vi "ClimbExecute.vi"(8 "error in (no error)":errorcluster) -> (0 "error out":errorcluster)   [LabVIEW 2023]
uses:
  <vilib>/Rock Robotics/WPI/ThirdParty/JAS_Junk/TrajLib/VI/BoolCmd_Recv_Internal.vi
  <vilib>/Rock Robotics/WPI/ThirdParty/JAS_Junk/TrajLib/VI/BoolCmd_ObtainQueue.vi
  <vilib>/Rock Robotics/Network Tables/NT Write Number.vi
  <vilib>/Rock Robotics/Network Tables/NT Write Boolean.vi
  <vilib>/Rock Robotics/WPI/ThirdParty/JAS_Junk/TrajLib/Trajectory_Library.lvlib
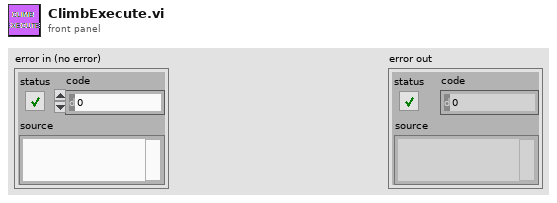
[diagram p1: front panel]
types:
  T1 = typedef "WPI_MotorControlDeviceRef.ctl" = cluster{"DeviceStatus":errorcluster, "Type":T2, "PWM":cluster{"PWM Channel":T3, "DeadBand":T4}, "CAN":cluster{"Device Number":u8, "SetOutput VI Ref":variant, "GetOutput VI Ref":variant, "Enable VI Ref":variant, "Disable VI Ref":variant, "Data":variant}, "Invert":bool, "DIO PWM":cluster{"PWM \"Enable\" Channel":T3, "DIOChannel":T5, "PWM Rate":dbl}}
  T2 = typedef "WPI_MotorControlType.ctl" = enum16{"PWM", "CAN", "DIO PWM"}
  T3 = typedef "FPGA_DIOPWMChannel.ctl" = enum8{"PWM 0", "PWM 1", "PWM 2", "PWM 3", "PWM 4", "PWM 5", "PWM 6", "PWM 7", "PWM 8", "PWM 9", "PWM MXP 0", "PWM MXP 1", "PWM MXP 2", "PWM MXP 3", "PWM MXP 4", "PWM MXP 5", "PWM MXP 6", "PWM MXP 7", "PWM MXP 8", "PWM MXP 9", "Invalid"}
  T4 = typedef "WPI_PWMDeadband.ctl" = cluster{"Name":string, "maxPositivePwm":i32, "minPositivePwm":i32, "centerPwm":i32, "maxNegativePwm":i32, "minNegativePwm":i32, "angularRange":u16}
  T5 = typedef "FPGA_DIOChannel.ctl" = enum8{"DIO 0", "DIO 1", "DIO 2", "DIO 3", "DIO 4", "DIO 5", "DIO 6", "DIO 7", "DIO 8", "DIO 9", "DIO MXP 0", "DIO MXP 1", "DIO MXP 2", "DIO MXP 3", "DIO MXP 4", "DIO MXP 5", "DIO MXP 6", "DIO MXP 7", "DIO MXP 8", "DIO MXP 9", "DIO MXP 10", "DIO MXP 11", "DIO MXP 12", "DIO MXP 13", "DIO MXP 14", "DIO MXP 15", "SPI Port CS1", "SPI Port CS2", "SPI Port CS3", "SPI Port MISO", "SPI Port MOSI", "Invalid"}
  T6 = typedef "Trajectory_Library.lvlib/PosCtrl_Tuning_Type.ctl" = cluster{"Slope":dbl, "Offset":dbl, "Error Deadband":dbl, "At Reference Count":i32, "Negate Output":bool, "Max Allowd Position":dbl, "Min Allowd Position":dbl}
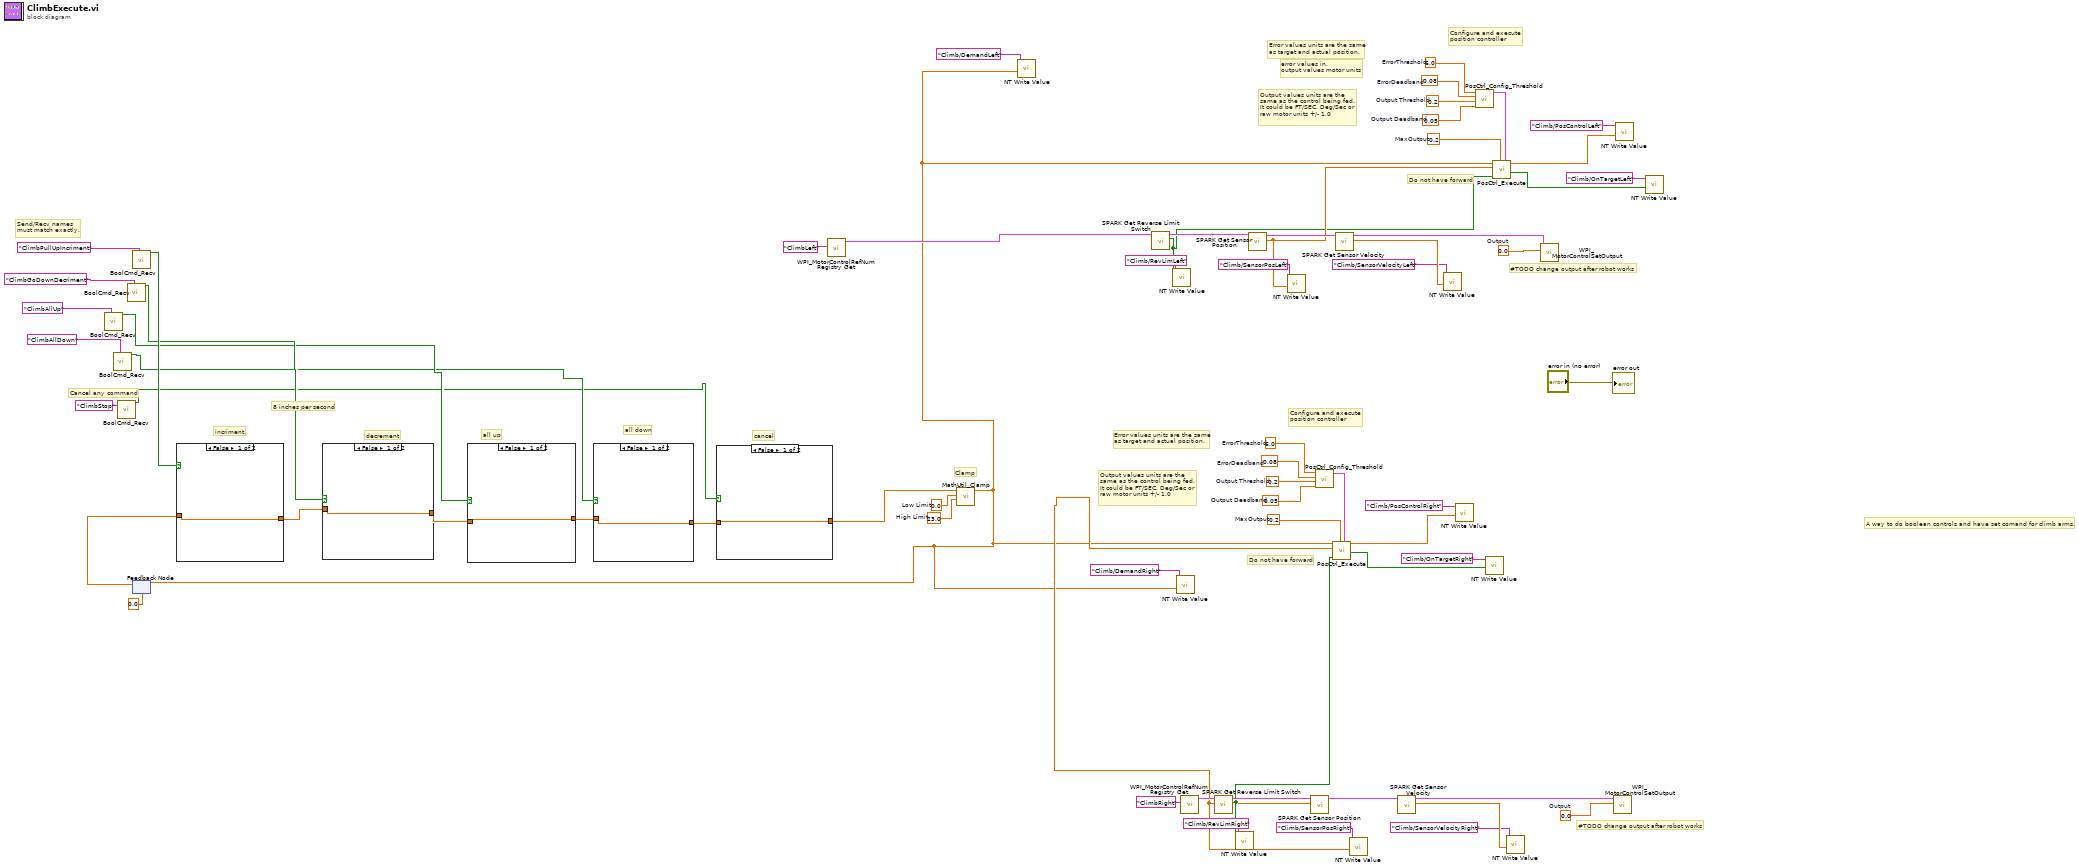
[diagram p0: block diagram]
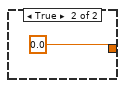
[diagram p3: hidden frame]
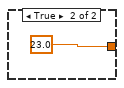
[diagram p4: hidden frame]
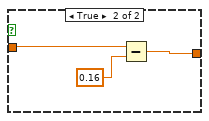
[diagram p5: hidden frame]
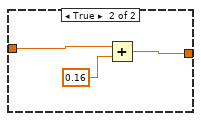
[diagram p6: hidden frame]
diagram:
  w12 = 23.0  # High Limit
  w11 = 0.0  # Low Limit
  w24 = 0.0  # Output
  w36 = 0.2  # MaxOutput
  w34 = 6.0  # ErrorThreshold
  w33 = 0.08  # ErrorDeadband
  w32 = 0.2  # Output Threshold
  w31 = 0.05  # Output Deadband
  w42 = 0.0  # Output
  w67 = 0.2  # MaxOutput
  w65 = 6.0  # ErrorThreshold
  w64 = 0.08  # ErrorDeadband
  w63 = 0.2  # Output Threshold
  w62 = 0.05  # Output Deadband
  # "cancel"
  # "Clamp"
  # "8 inches per second"
  # "all down"
  # "all up"
  # "decrement"
  # "incriment"
  # "Cancel any command"
  # "Send/Recv names\nmust match exactly."
  # "A way to do boolean controls and have set comand for climb arms."
  # "error values in.\noutput values motor units"
  # "#TODO change output after robot works"
  # "Do not have forward"
  # "Output values units are the\nsame as the control being fed.  \nIt could be FT/SEC, Deg/Sec or\nraw motor units +/- 1.0"
  # "Error values units are the same \nas target and actual position."
  # "Configure and execute \nposition controller"
  # "#TODO change output after robot works"
  # "Do not have forward"
  # "Output values units are the\nsame as the control being fed.  \nIt could be FT/SEC, Deg/Sec or\nraw motor units +/- 1.0"
  # "Error values units are the same \nas target and actual position."
  # "Configure and execute \nposition controller"
  n1 = call <vilib>:"BoolCmd_Recv.vi"("Command Name"="ClimbAllUp") -> ("New Request"=w4:bool)  [unwired: 9 in, 1 out]
  n2 = call <vilib>:"BoolCmd_Recv.vi"("Command Name"="ClimbAllDown") -> ("New Request"=w3:bool)  [unwired: 9 in, 1 out]
  n3 = call <vilib>:"BoolCmd_Recv.vi"("Command Name"="ClimbStop") -> ("New Request"=w2:bool)  [unwired: 9 in, 1 out]
  n4 = call <vilib>:"BoolCmd_Recv.vi"("Command Name"="ClimbGoDownDecriment") -> ("New Request"=w5:bool)  [unwired: 9 in, 1 out]
  n5 = call <vilib>:"BoolCmd_Recv.vi"("Command Name"="ClimbPullUpIncriment") -> ("New Request"=w6:bool)  [unwired: 9 in, 1 out]
  n6 = feedback #1(0.0 ("false")) -> (w16:dbl)
  n7 = case shown="False" w6 {
    tunnel: w16 -> [w68 w71]
    tunnel: [w68 w69] -> w15
    frame False {
    }
    frame True {
      n8 = Add(x=w71, y=0.16) -> (x+y=w69:dbl)
    }
  }
  n9 = case shown="False" w5 {
    tunnel: w15 -> [w72 w74]
    tunnel: [w72 w73] -> w14
    frame False {
    }
    frame True {
      n10 = Subtract(x=w74, y=0.16) -> (x-y=w73:dbl)
    }
  }
  n11 = case shown="False" w4 {
    tunnel: w14 -> [w76 _]
    tunnel: [w76 23.0 ("y")] -> w13
    frame False {
    }
    frame True {
    }
  }
  n12 = case shown="False" w3 {
    tunnel: w13 -> [w78 _]
    tunnel: [w78 0.0 ("y")] -> w8
    frame False {
    }
    frame True {
    }
  }
  n13 = case shown="False" w2 {
    tunnel: w8 -> [w80 w81]
    tunnel: [w80 w81] -> w7
    frame False {
    }
    frame True {
    }
  }
  n14 = call <vilib>:"WPI_MotorControlRefNum Registry Get.vi"("refnum name"="ClimbLeft") -> ("MotorControlDevRef"=w61:T1)  [unwired: 9 in, 1 out]
  n15 = call <vilib>:"MathUtil_Clamp.vi"("High Limit"=w12, "Low Limit"=w11, "Value"=w7) -> ("Result"=w9:dbl)  [unwired: 8 in]
  n16 = feedback-in #1(w9) -> ()
  n17 = call-poly <vilib>:"NT Write Value.vi"("value"=w9, "name"="Climb/DemandLeft") -> ()  [unwired: 9 in, 1 out]
  n18 = call <vilib>:"SPARK Get Reverse Limit Switch.vi"("MotorControlDevRef in"=w61) -> ("Hard Limit Rev"=w44:bool, "MotorControlDevRef out"=w58:T1)  [unwired: 7 in, 2 out]
  n19 = call-poly <vilib>:"NT Write Value.vi"("value"=w44, "name"="Climb/RevLimLeft") -> ()  [unwired: 9 in, 1 out]
  n20 = call-poly <vilib>:"NT Write Value.vi"("value"=w9, "name"="Climb/DemandRight") -> ()  [unwired: 9 in, 1 out]
  n21 = call <vilib>:"WPI_MotorControlRefNum Registry Get.vi"("refnum name"="ClimbRight") -> ("MotorControlDevRef"=w53:T1)  [unwired: 9 in, 1 out]
  n22 = call <vilib>:"SPARK Get Reverse Limit Switch.vi"("MotorControlDevRef in"=w53) -> ("Hard Limit Rev"=w26:bool, "MotorControlDevRef out"=w50:T1)  [unwired: 7 in, 2 out]
  n23 = call-poly <vilib>:"NT Write Value.vi"("value"=w26, "name"="Climb/RevLimRight") -> ()  [unwired: 9 in, 1 out]
  n24 = call <vilib>:"SPARK Get Sensor Position.vi"("MotorControlDevRef in"=w58) -> ("Sensor Position"=w45:dbl, "MotorControlDevRef out"=w60:T1)  [unwired: 7 in, 2 out]
  n25 = call-poly <vilib>:"NT Write Value.vi"("value"=w45, "name"="Climb/SensorPosLeft") -> ()  [unwired: 9 in, 1 out]
  n26 = call <vilib>:"SPARK Get Sensor Position.vi"("MotorControlDevRef in"=w50) -> ("Sensor Position"=w10:dbl, "MotorControlDevRef out"=w52:T1)  [unwired: 7 in, 2 out]
  n27 = call <vilib>:"PosCtrl_Config_Threshold.vi"("Output Deadband"=w31, "Output Threshold"=w32, "ErrorDeadband"=w33, "ErrorThreshold"=w34) -> ("PosCtrl_Config_Params"=w35:T6)  [unwired: 7 in]
  n28 = call <vilib>:"PosCtrl_Execute.vi"("PosCtrl_Config_Params"=w35, "MaxOutput"=w36, "Rev Limit Switch"=w26, "CurrentPosition"=w10, "TargetPosition"=w9) -> ("OnTarget"=w28:bool, "Output"=w29:dbl)  [unwired: 4 in, 1 out]
  n29 = call <vilib>:"SPARK Get Sensor Velocity.vi"("MotorControlDevRef in"=w60) -> ("Sensor Velocity"=w55:dbl, "MotorControlDevRef out"=w43:T1)  [unwired: 7 in, 2 out]
  n30 = call-poly <vilib>:"NT Write Value.vi"("value"=w10, "name"="Climb/SensorPosRight") -> ()  [unwired: 9 in, 1 out]
  n31 = call <vilib>:"SPARK Get Sensor Velocity.vi"("MotorControlDevRef in"=w52) -> ("Sensor Velocity"=w47:dbl, "MotorControlDevRef out"=w23:T1)  [unwired: 7 in, 2 out]
  n32 = call-poly <vilib>:"NT Write Value.vi"("value"=w55, "name"="Climb/SensorVelocityLeft") -> ()  [unwired: 9 in, 1 out]
  n33 = call-poly <vilib>:"NT Write Value.vi"("value"=w29, "name"="Climb/PosControlRight") -> ()  [unwired: 9 in, 1 out]
  n34 = call <vilib>:"PosCtrl_Config_Threshold.vi"("Output Deadband"=w62, "Output Threshold"=w63, "ErrorDeadband"=w64, "ErrorThreshold"=w65) -> ("PosCtrl_Config_Params"=w66:T6)  [unwired: 7 in]
  n35 = call-poly <vilib>:"NT Write Value.vi"("value"=w28, "name"="Climb/OnTargetRight") -> ()  [unwired: 9 in, 1 out]
  n36 = call <vilib>:"PosCtrl_Execute.vi"("PosCtrl_Config_Params"=w66, "MaxOutput"=w67, "Rev Limit Switch"=w44, "CurrentPosition"=w45, "TargetPosition"=w9) -> ("OnTarget"=w38:bool, "Output"=w40:dbl)  [unwired: 4 in, 1 out]
  n37 = call-poly <vilib>:"NT Write Value.vi"("value"=w47, "name"="Climb/SensorVelocityRight") -> ()  [unwired: 9 in, 1 out]
  n38 = call <vilib>:"WPI_MotorControlSetOutput.vi"("Output"=w42, "MotorControlDevRef"=w43) -> ()  [unwired: 7 in, 3 out]
  n39 = call <vilib>:"WPI_MotorControlSetOutput.vi"("Output"=w24, "MotorControlDevRef"=w23) -> ()  [unwired: 7 in, 3 out]
  n40 = call-poly <vilib>:"NT Write Value.vi"("value"=w40, "name"="Climb/PosControlLeft") -> ()  [unwired: 9 in, 1 out]
  n41 = call-poly <vilib>:"NT Write Value.vi"("value"=w38, "name"="Climb/OnTargetLeft") -> ()  [unwired: 9 in, 1 out]
  "error out" <- "error in (no error)"
